vi "Set Server State.vi"(8 "error in (no error)":errorcluster, 10 "New State":T1, 11 "Template Server in":refnum<class "OCV2.lvclass">) -> (0 "error out":errorcluster, 2 "Previous State":T1, 3 "Template Server out":refnum<class "OCV2.lvclass">)   [LabVIEW 2019, in "OCV2.lvlib" / "OCV2.lvclass"]
uses:
  OCV2.lvclass
  typeDefs/Server State Data.ctl
  OCV2.lvclass/OCV2.ctl
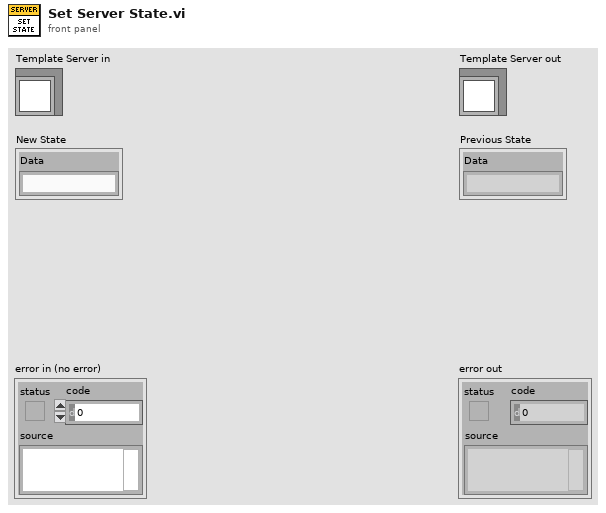
[diagram p1: front panel]
types:
  T1 = typedef "OCV2.lvlib/OCV2.lvclass/Server State Data.ctl" = cluster{"Data":string}
  T2 = typedef "Template Server.lvlib/Template Server.lvclass/Server State Data.ctl" = cluster{"Data":string}
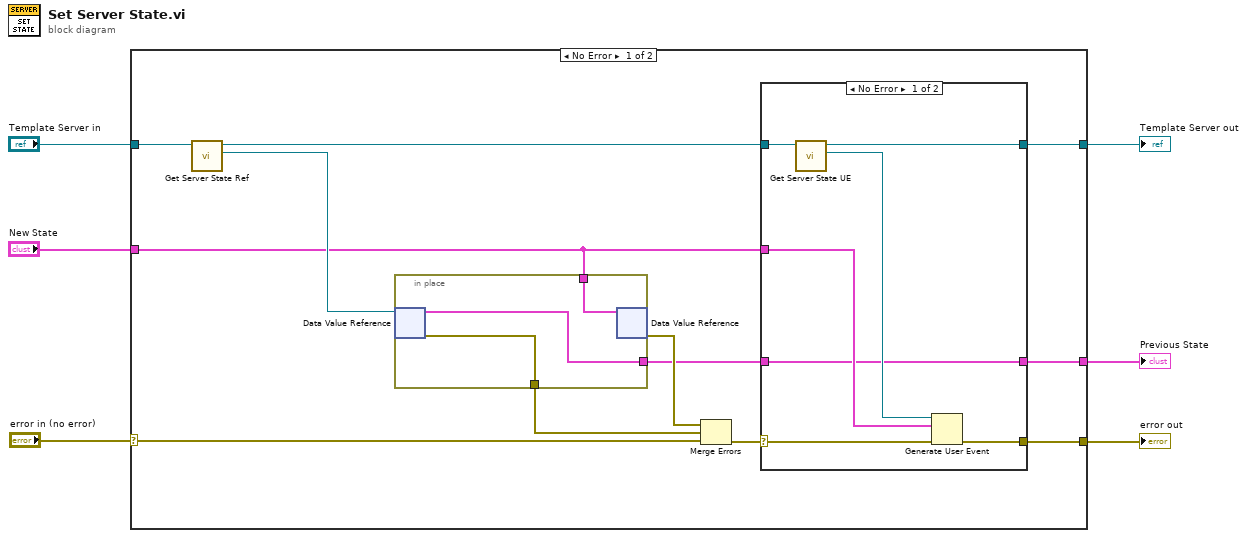
[diagram p0: block diagram]
diagram:
  n1 = case shown="No Error" "error in (no error)" {
    selector: "error in (no error)" -> [w16 w33]
    tunnel: [w11 w33] -> w5
    tunnel: [w10 w32] -> w3
    tunnel: "Template Server in" -> [w18 w32]
    tunnel: "New State" -> [w9 _]
    tunnel: [w7 _] -> w1
    frame No Error {
      n2 = call "Get Server State Ref.vi"("Template Server in"=w18) -> ("Server State Ref"=w17:refnum<data-value>, "Template Server out"=w13:refnum<class "OCV2.lvclass">)  [unwired: 9 in]
      n3 = in-place {
        in-place-border: w9 -> [w31]
        in-place-border: [w30] -> w8
        in-place-border: [w29] -> w15
        n4 = in-place-dvr #1(w17) -> (w30:T2, w29:errorcluster)
        n5 = in-place-dvr #1(w31) -> (w14:errorcluster)  [unwired: 1 out]
      }
      n6 = Merge Errors(w14, w15, w16) -> (w12:errorcluster)
      n7 = case shown="No Error" w12 {
        selector: w12 -> [w23 w28]
        tunnel: w13 -> [w25 w27]
        tunnel: [w22 w28] -> w11
        tunnel: [w24 w27] -> w10
        tunnel: w9 -> [w20 _]
        tunnel: w8 -> [w19 w26]
        tunnel: [w19 w26] -> w7
        frame No Error {
          n8 = call "Get Server State UE.vi"("Template Server in"=w25) -> ("Server Internal State UE"=w21:refnum<user-event>, "Template Server out"=w24:refnum<class "OCV2.lvclass">)  [unwired: 9 in]
          n9 = Generate User Event(user event=w21, event data cluster=w20, error in=w23) -> (error out=w22:errorcluster)  [unwired: 1 in, 1 out]
        }
        frame Error {
        }
      }
    }
    frame Error {
    }
  }
  "error out" <- w5
  "Template Server out" <- w3
  "Previous State" <- w1
